vi "googlescript.vi"() -> ()   [LabVIEW 2016]
uses:
  <vilib>/httpClient/LabVIEWHTTPClient.lvlib
panel:
  in  "stop":bool
  out "Full URL":string
  in  "Foneyvalue":dbl(slide) scale=0.0..10.0
  in  "Moneyvalue":dbl(slide) scale=0.0..10.0
  in  "Concat":string="https://script.google.com/macros/s/AKfycbxFw-vYWsMeyY0yPKPZr-sJ4ZorYB6e1rczfIqwViIpXXHFbn3u/exec?"
  in  "foney":string="https://script.google.com/macros/s/AKfycbxFw-vYWsMeyY0yPKPZr-sJ4ZorYB6e1rczfIqwViIpXXHFbn3u/exec?"
  in  "money":string="https://script.google.com/macros/s/AKfycbxFw-vYWsMeyY0yPKPZr-sJ4ZorYB6e1rczfIqwViIpXXHFbn3u/exec?"
  in  "String":string="https://script.google.com/macros/s/AKfycbxFw-vYWsMeyY0yPKPZr-sJ4ZorYB6e1rczfIqwViIpXXHFbn3u/exec?"
  # "Daniel Smith de Paz"
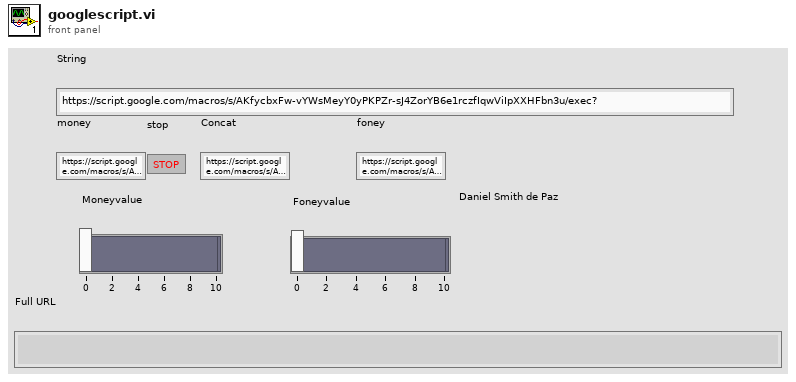
[diagram p1: front panel]
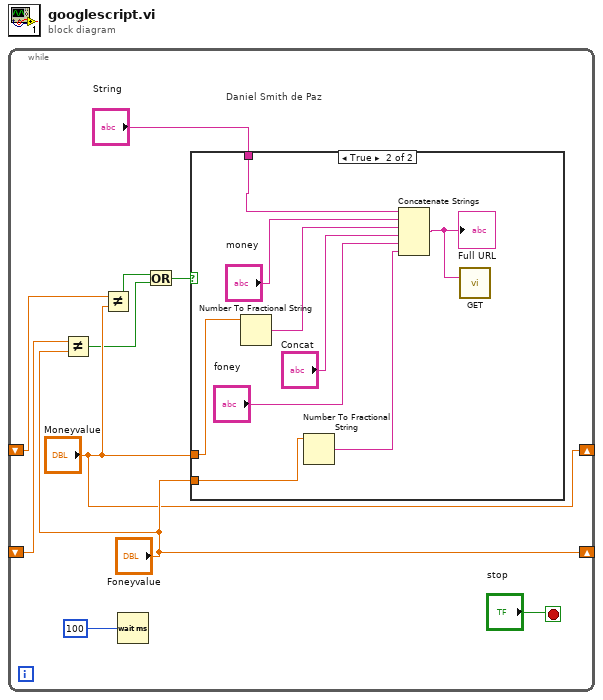
[diagram p0: block diagram]
diagram:
  n1 = while {
    shift-right: ["Foneyvalue"] -> _
    shift-left: _ -> [w7]
    shift-right: ["Moneyvalue"] -> _
    shift-left: _ -> [w5]
    stop <- "stop" stop-if-true
    # "Daniel Smith de Paz"
    n2 = Not Equal?(x=w7, y="Foneyvalue") -> (x != y?=w3:bool)
    n3 = Not Equal?(x=w5, y="Moneyvalue") -> (x != y?=w2:bool)
    n4 = Wait (ms)(milliseconds to wait=u32 100) -> ()  [unwired: 1 out]
    n5 = Or(x=w2, y=w3) -> (x .or. y?=w4:bool)
    n6 = case shown="True" w4 {
      tunnel: "String" -> [_ w19]
      tunnel: "Moneyvalue" -> [_ w17]
      tunnel: "Foneyvalue" -> [_ w13]
      frame False {
      }
      frame True {
        n7 = Number To Fractional String(number=w17) -> (F-format string=w16:string)  [unwired: 3 in]
        n8 = Number To Fractional String(number=w13) -> (F-format string=w12:string)  [unwired: 3 in]
        n9 = Concatenate Strings(w19, "money", w16, "Concat", "foney", w12) -> (w11:string)
        "Full URL" <- w11
        n10 = call <vilib>:"GET.vi"("url"=w11) -> ()  [unwired: 11 in, 4 out]
      }
    }
  }
